vi "Overlay Points with User Specified Size.vi"(6 "Color":u32(colorbox)=16711680, 7 "Group":string, 8 "error in":errorcluster, 9 "Point Diameter (5)":u32=5 min=3 max=1000, 10 "Points":cluster{"X":i32, "Y":i32}[](array[cluster]), 11 "Image In":T1) -> (0 "error out":errorcluster, 3 "Image Out":T1)   [LabVIEW 2018]
doc: "Overlay an array of points with user specified radius of dots."
uses:
  <vilib>/vision/Image Controls.llb/IMAQ Image.ctl
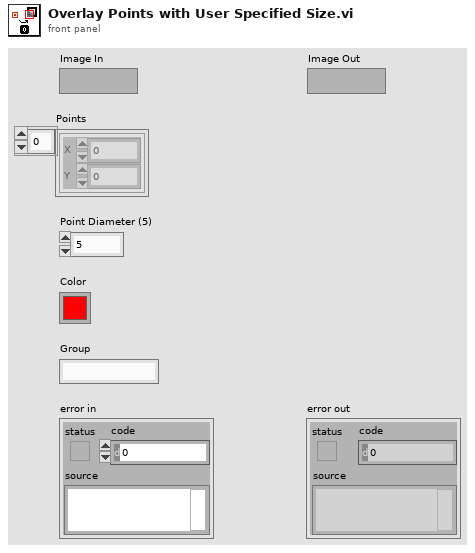
[diagram p1: front panel]
types:
  T1 = typedef "IMAQ Image.ctl" = refnum<image>
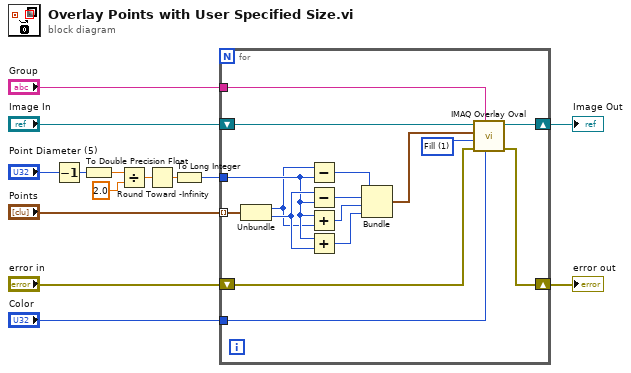
[diagram p0: block diagram]
diagram:
  n1 = Decrement(x="Point Diameter (5)") -> (x-1=w13:u32)
  n2 = To Double Precision Float(number=w13) -> (double precision float=w4:dbl)
  n3 = Divide(x=w4, y=2.0) -> (x/y=w9:dbl)
  n4 = Round Toward -Infinity(1:w9) -> (0:w11:dbl)
  n5 = To Long Integer(number=w11) -> (32bit integer=w2:i32)
  n6 = for {
    tunnel: "Points" -> [w30] mode=indexing
    tunnel: w2 -> [w27]
    tunnel: "Color" -> [w20]
    tunnel: "Group" -> [w18]
    shift-right: [w17] -> w6
    shift-left: "Image In" -> [w29]
    shift-right: [w15] -> w1
    shift-left: "error in" -> [w19]
    w16 = u32 1 items=["Frame", "Fill"] ("Drawing Mode (Frame)")
    n7 = Unbundle(w30) -> ("X"=w26:i32, "Y"=w28:i32)
    n8 = Subtract(x=w26, y=w27) -> (x-y=w25:i32)
    n9 = Subtract(x=w28, y=w27) -> (x-y=w24:i32)
    n10 = Add(x=w27, y=w26) -> (x+y=w23:i32)
    n11 = Add(x=w27, y=w28) -> (x+y=w22:i32)
    n12 = Bundle(w25, w24, w23, w22) -> (w21:cluster{i32, i32, i32, i32})  [unwired: 1 in]
    n13 = call "IMAQ Overlay Oval"("Color"=w20, "Group"=w18, "error in (no error)"=w19, "Drawing Mode (Frame)"=w16, "Bounding Rectangle"=w21, "Image"=w29) -> ("error out"=w15:errorcluster, "Image Out"=w17:T1)  [unwired: 4 in]
  }
  "Image Out" <- w6
  "error out" <- w1
